vi "Read Max Min.vi"(0 "VISA resource name":refnum<visa-resource-name>, 11 "error in (no error)":errorcluster) -> (3 "Measurement Count":dbl, 4 "VISA resource name out":refnum<visa-resource-name>, 6 "Maximum Value":dbl, 8 "Average Value":dbl, 10 "Minimum Value":dbl, 14 "Total Value":dbl, 15 "error out":errorcluster)   [LabVIEW 2017, in "ADCMT 6240.lvlib"]
doc: "Queries the result of Max/Min calculation.\nBefore use this VI, you must enable calculate Max and Min."
uses:
  ADCMT 6240.lvlib
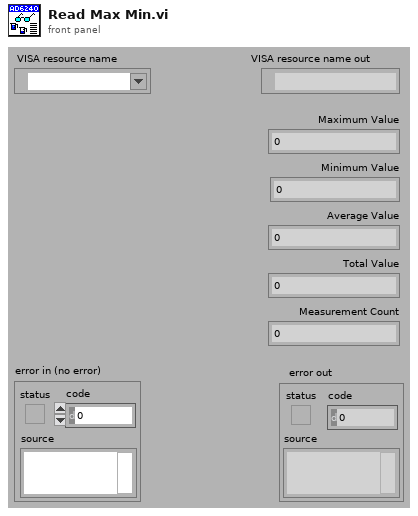
[diagram p1: front panel]
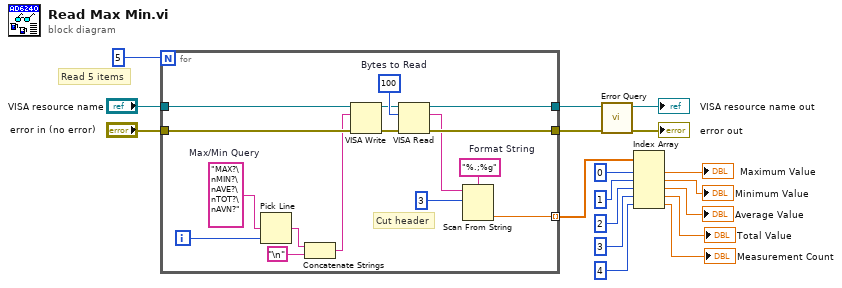
[diagram p0: block diagram]
diagram:
  # "Read 5 items"
  n1 = for "Forループ" {
    N: 5 -> [_]
    tunnel: "VISA resource name" -> [w34]
    tunnel: [w30] -> w17
    tunnel: [w29] -> w16
    tunnel: "error in (no error)" -> [w28]
    tunnel: [w23] -> w10 mode=indexing
    i -> [w24]
    w25 = "MAX?\nMIN?\nAVE?\nTOT?\nAVN?"  # Max/Min Query
    w27 = "%.;%g"  # Format String
    w33 = u32 100  # Bytes to Read
    # "Cut header"
    n2 = Pick Line ("ライン選択")(multi-line string=w25, line index=w24) -> (output string=w20:string)  [unwired: 1 in]
    n3 = Concatenate Strings(w20, "\n") -> (w19:string)
    n4 = VISA Write ("VISA書き込み")(VISA resource name=w34, write buffer=w19, error in (no error)=w28) -> (VISA resource name out=w32:refnum<visa-resource-name>, error out=w31:errorcluster)  [unwired: 1 out]
    n5 = VISA Read ("VISA読み取り")(VISA resource name=w32, byte count=w33, error in (no error)=w31) -> (VISA resource name out=w29:refnum<visa-resource-name>, read buffer=w26:string, error out=w30:errorcluster)  [unwired: 1 out]
    n6 = Scan From String ("文字列からスキャン")(format string=w27, input string=w26, initial scan location=3) -> (output 1=w23:dbl)  [unwired: 2 in, 3 out]
  }
  n7 = call "Error Query.vi"("error in (no error)"=w17, "VISA resource name"=w16) -> ("error out"=→"error out":errorcluster, "VISA resource name out"=→"VISA resource name out":refnum<visa-resource-name>)  [unwired: 6 in, 2 out]
  n8 = Index Array(array=w10, index #1=0, index #2=1, index #3=2, index #4=3, index #5=4) -> (element #1=→"Maximum Value":dbl, element #2=→"Minimum Value":dbl, element #3=→"Average Value":dbl, element #4=→"Total Value":dbl, element #5=→"Measurement Count":dbl)
